vi "WS6-600- Main v0.1.vi"() -> ()   [LabVIEW 2017]
uses:
  wlmData.dll
  <vilib>/Analysis/NI_AALBase.lvlib
panel:
  in  "stop":bool
  out "mean":dbl format="%0.2f"
  out "Waveform Chart":dbl(graph)
  in  "W6 Shots to Average":i32=10
  out "GetMaxPeak(0)":i16
  out "GetMinPeak(0)":i16
  out "GetExposure2(0)":u16 format="%.0f ms"
  out "GetExposure(0)":u16 format="%.0f ms"
  out "Instantiate(0, RM, 0, 0)":u32
  in  "RM":i32 min=0 max=1 step=1
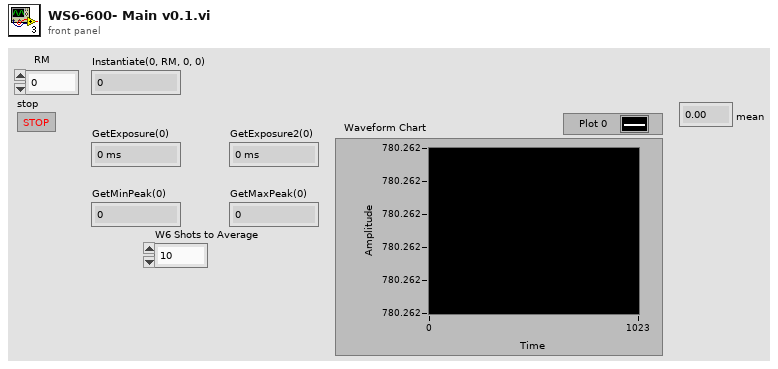
[diagram p1: front panel]
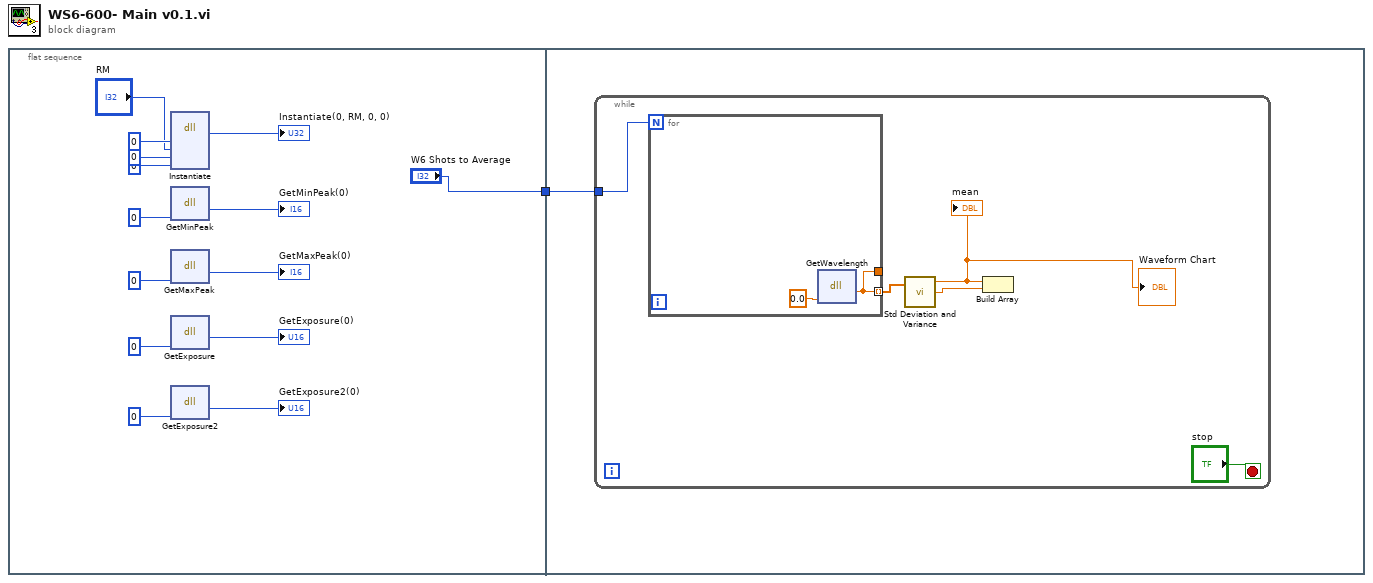
[diagram p0: block diagram]
diagram:
  n1 = flat-sequence {
    tunnel: ["W6 Shots to Average"] -> w1
    tunnel: w1 -> [w16]
    frame #0 {
      n2 = dll-call lib="wlmData.dll" fn="Instantiate"("arg1"=u32 0, "arg2"="RM", "arg3"=u32 0, "arg4"=u32 0) -> ("return type"=→"Instantiate(0, RM, 0, 0)":u32)  [unwired: 7 in, 2 out]
      n3 = dll-call lib="wlmData.dll" fn="GetMinPeak"("arg1"=0) -> ("return type"=→"GetMinPeak(0)":i32)  [unwired: 4 in, 2 out]
      n4 = dll-call lib="wlmData.dll" fn="GetMaxPeak"("arg1"=0) -> ("return type"=→"GetMaxPeak(0)":i32)  [unwired: 4 in, 2 out]
      n5 = dll-call lib="wlmData.dll" fn="GetExposure"("arg1"=0) -> ("return type"=→"GetExposure(0)":i32)  [unwired: 4 in, 2 out]
      n6 = dll-call lib="wlmData.dll" fn="GetExposure2"("arg1"=0) -> ("return type"=→"GetExposure2(0)":i32)  [unwired: 4 in, 2 out]
    }
    frame #1 {
      n7 = while {
        tunnel: w16 -> [w21]
        stop <- "stop" stop-if-true
        n8 = for {
          N: w21 -> [_]
          tunnel: [w22] -> w20 mode=indexing
          tunnel: [w22] -> _
          n9 = dll-call lib="wlmData.dll" fn="GetWavelength"("arg1"=0.0) -> ("return type"=w22:dbl)  [unwired: 4 in, 2 out]
        }
        n10 = call <vilib>:"Std Deviation and Variance.vi"("X"=w20) -> ("mean"=w17:dbl, "standard deviation"=w19:dbl)  [unwired: 1 in, 1 out]
        "mean" <- w17
        "Waveform Chart" <- w17
        n11 = Build Array(w17, w19) -> ()  [unwired: 1 out]
      }
    }
  }
